vi "Get RLC Circuit Frequency Responce.vi"(0 "Vin amplitude":dbl=240.0 format="%0.2f", 1 "Circuit Type Enum":T2, 5 "Resistence (R)":dbl=10.0, 7 "Impedence (H)":dbl=0.01, 9 "Capacitave (F)":dbl=7.5e-06, 11 "error in (no error)":errorcluster) -> (3 "Frequency Response Picture":picture, 4 "Frequency Response Image Data":T1, 14 "Frequency Response":cluster{"X":dbl[], "Y":dbl[]}[](graph)=[{"X"=[0.0, 1.0, 2.0, 3.0, 4.0, 5.0, 6.0, 7.0, 8.0, 9.0, 10.0, 11.0, 12.0, 13.0, 14.0, 15.0, 16.0, 17.0, 18.0, 19.0, 20.0, 21.0, 22.0, 23.0, 24.0, 25.0, 26.0, 27.0, 28.0, 29.0, 30.0, 31.0, 32.0, 33.0, 34.0, 35.0, 36.0, 37.0, 38.0, 39.0, 40.0, 41.0, 42.0, 43.0, 44.0, 45.0, 46.0, 47.0, 48.0, 49.0, 50.0, 51.0, 52.0, 53.0, 54.0, 55.0, 56.0, 57.0, 58.0, 59.0, 60.0, 61.0, 62.0, 63.0, 64.0, 65.0, 66.0, 67.0, 68.0, 69.0, 70.0, 71.0, 72.0, 73.0, 74.0, 75.0, 76.0, 77.0], "Y"=[0.0, 0.0001279093439907941, 0.0005116286274565821, 0.0011511316053372826, 0.002046374537398417, 0.003197296190529561, 0.004603817841962096, 0.006265843283406199, 0.008183258826106956, 0.010355933306819496, 0.012783718094703, 0.01546644709913344, 0.018403936778434823, 0.0215959861495288, 0.025042376798502308, 0.028742872892093246, 0.0326972211900935, 0.036905151058669455, 0.04136637448459942, 0.04608058609042774, 0.05104746315053532, 0.05626666560812573, 0.061737836093127274, 0.06746059994101006, 0.07343456521251747, 0.07965932271431238, 0.08613444602053646, 0.09285949149528333, 0.09983399831598429, 0.10705748849770579, 0.11452946691835893, 0.12224942134482022, 0.13021682245996197, 0.13843112389059317, 0.14689176223630918, 0.1555981570992499, 0.164549711114766, 0.17374580998299163, 0.18318582250132406, 0.19286910059780862, 0.2027949793654282, 0.21296277709729705, 0.22337179532275803, 0.2340213188443811, 0.24491061577586495, 0.2560389375808376, 0.2674055191125576, 0.279009578654514, 0.2908503179619234, 0.3029269223041252, 0.3152385605078709, 0.3277843850015102, 0.3405635318600694, 0.35357512085122345, 0.36681825548215957, 0.38029202304733173, 0.39399549467710293, 0.40792772538727934, 0.4220877541295284, 0.43647460384268355, 0.4510872815049364, 0.46592477818690975, 0.48098606910561315, 0.49627011367928237, 0.5117758555830951, 0.5275022228057681, 0.5434481277070307, 0.5596124670759731, 0.5759941221902721, 0.5925919588762874, 0.6094048275700303, 0.6264315633790047, 0.6436709861449139, 0.6611219005072388, 0.6787830959676776, 0.6966533469554558, 0.7147314128934922, 0.7330160382654349]}, {"X"=[581.1516831325472, 581.1516831325472, 581.1516831325472, 581.1516831325472, 581.1516831325472, 581.1516831325472, 581.1516831325472, 581.1516831325472, 581.1516831325472, 581.1516831325472, 581.1516831325472, 581.1516831325472, 581.1516831325472, 581.1516831325472, 581.1516831325472, 581.1516831325472, 581.1516831325472, 581.1516831325472, 581.1516831325472, 581.1516831325472, 581.1516831325472, 581.1516831325472, 581.1516831325472, 581.1516831325472, 581.1516831325472, 581.1516831325472, 581.1516831325472, 581.1516831325472, 581.1516831325472, 581.1516831325472, 581.1516831325472, 581.1516831325472, 581.1516831325472, 581.1516831325472, 581.1516831325472, 581.1516831325472, 581.1516831325472, 581.1516831325472, 581.1516831325472, 581.1516831325472, 581.1516831325472, 581.1516831325472, 581.1516831325472, 581.1516831325472, 581.1516831325472, 581.1516831325472, 581.1516831325472, 581.1516831325472, 581.1516831325472, 581.1516831325472, 581.1516831325472, 581.1516831325472, 581.1516831325472, 581.1516831325472, 581.1516831325472, 581.1516831325472, 581.1516831325472, 581.1516831325472, 581.1516831325472, 581.1516831325472, 581.1516831325472, 581.1516831325472, 581.1516831325472, 581.1516831325472, 581.1516831325472, 581.1516831325472, 581.1516831325472, 581.1516831325472, 581.1516831325472, 581.1516831325472, 581.1516831325472, 581.1516831325472, 581.1516831325472, 581.1516831325472, 581.1516831325472, 581.1516831325472, 581.1516831325472, 581.1516831325472], "Y"=[0.0, 0.0, 0.0, 0.0, 0.0, 0.0, 0.0, 0.0, 0.0, 0.0, 0.0, 0.0, 0.0, 0.0, 0.0, 0.0, 0.0, 0.0, 0.0, 0.0, 0.0, 0.0, 0.0, 0.0, 0.0, 0.0, 0.0, 0.0, 0.0, 0.0, 0.0, 0.0, 0.0, 0.0, 0.0, 0.0, 0.0, 0.0, 0.0, 0.0, 0.0, 0.0, 0.0, 0.0, 0.0, 0.0, 0.0, 0.0, 0.0, 0.0, 0.0, 0.0, 0.0, 0.0, 0.0, 0.0, 0.0, 0.0, 0.0, 0.0, 0.0, 0.0, 0.0, 0.0, 0.0, 0.0, 0.0, 0.0, 0.0, 0.0, 0.0, 0.0, 0.0, 0.0, 0.0, 0.0, 0.0, 0.0]}, {"X"=[290.5758415662736, 290.5758415662736, 290.5758415662736, 290.5758415662736, 290.5758415662736, 290.5758415662736, 290.5758415662736, 290.5758415662736, 290.5758415662736, 290.5758415662736, 290.5758415662736, 290.5758415662736, 290.5758415662736, 290.5758415662736, 290.5758415662736, 290.5758415662736, 290.5758415662736, 290.5758415662736, 290.5758415662736, 290.5758415662736, 290.5758415662736, 290.5758415662736, 290.5758415662736, 290.5758415662736, 290.5758415662736, 290.5758415662736, 290.5758415662736, 290.5758415662736, 290.5758415662736, 290.5758415662736, 290.5758415662736, 290.5758415662736, 290.5758415662736, 290.5758415662736, 290.5758415662736, 290.5758415662736, 290.5758415662736, 290.5758415662736, 290.5758415662736, 290.5758415662736, 290.5758415662736, 290.5758415662736, 290.5758415662736, 290.5758415662736, 290.5758415662736, 290.5758415662736, 290.5758415662736, 290.5758415662736, 290.5758415662736, 290.5758415662736, 290.5758415662736, 290.5758415662736, 290.5758415662736, 290.5758415662736, 290.5758415662736, 290.5758415662736, 290.5758415662736, 290.5758415662736, 290.5758415662736, 290.5758415662736, 290.5758415662736, 290.5758415662736, 290.5758415662736, 290.5758415662736, 290.5758415662736, 290.5758415662736, 290.5758415662736, 290.5758415662736, 290.5758415662736, 290.5758415662736, 290.5758415662736, 290.5758415662736, 290.5758415662736, 290.5758415662736, 290.5758415662736, 290.5758415662736, 290.5758415662736, 290.5758415662736], "Y"=[0.0, 0.0, 0.0, 0.0, 0.0, 0.0, 0.0, 0.0, 0.0, 0.0, 0.0, 0.0, 0.0, 0.0, 0.0, 0.0, 0.0, 0.0, 0.0, 0.0, 0.0, 0.0, 0.0, 0.0, 0.0, 0.0, 0.0, 0.0, 0.0, 0.0, 0.0, 0.0, 0.0, 0.0, 0.0, 0.0, 0.0, 0.0, 0.0, 0.0, 0.0, 0.0, 0.0, 0.0, 0.0, 0.0, 0.0, 0.0, 0.0, 0.0, 0.0, 0.0, 0.0, 0.0, 0.0, 0.0, 0.0, 0.0, 0.0, 0.0, 0.0, 0.0, 0.0, 0.0, 0.0, 0.0, 0.0, 0.0, 0.0, 0.0, 0.0, 0.0, 0.0, 0.0, 0.0, 0.0, 0.0, 0.0]}, {"X"=[871.7275246988208, 871.7275246988208, 871.7275246988208, 871.7275246988208, 871.7275246988208, 871.7275246988208, 871.7275246988208, 871.7275246988208, 871.7275246988208, 871.7275246988208, 871.7275246988208, 871.7275246988208, 871.7275246988208, 871.7275246988208, 871.7275246988208, 871.7275246988208, 871.7275246988208, 871.7275246988208, 871.7275246988208, 871.7275246988208, 871.7275246988208, 871.7275246988208, 871.7275246988208, 871.7275246988208, 871.7275246988208, 871.7275246988208, 871.7275246988208, 871.7275246988208, 871.7275246988208, 871.7275246988208, 871.7275246988208, 871.7275246988208, 871.7275246988208, 871.7275246988208, 871.7275246988208, 871.7275246988208, 871.7275246988208, 871.7275246988208, 871.7275246988208, 871.7275246988208, 871.7275246988208, 871.7275246988208, 871.7275246988208, 871.7275246988208, 871.7275246988208, 871.7275246988208, 871.7275246988208, 871.7275246988208, 871.7275246988208, 871.7275246988208, 871.7275246988208, 871.7275246988208, 871.7275246988208, 871.7275246988208, 871.7275246988208, 871.7275246988208, 871.7275246988208, 871.7275246988208, 871.7275246988208, 871.7275246988208, 871.7275246988208, 871.7275246988208, 871.7275246988208, 871.7275246988208, 871.7275246988208, 871.7275246988208, 871.7275246988208, 871.7275246988208, 871.7275246988208, 871.7275246988208, 871.7275246988208, 871.7275246988208, 871.7275246988208, 871.7275246988208, 871.7275246988208, 871.7275246988208, 871.7275246988208, 871.7275246988208], "Y"=[0.0, 0.0, 0.0, 0.0, 0.0, 0.0, 0.0, 0.0, 0.0, 0.0, 0.0, 0.0, 0.0, 0.0, 0.0, 0.0, 0.0, 0.0, 0.0, 0.0, 0.0, 0.0, 0.0, 0.0, 0.0, 0.0, 0.0, 0.0, 0.0, 0.0, 0.0, 0.0, 0.0, 0.0, 0.0, 0.0, 0.0, 0.0, 0.0, 0.0, 0.0, 0.0, 0.0, 0.0, 0.0, 0.0, 0.0, 0.0, 0.0, 0.0, 0.0, 0.0, 0.0, 0.0, 0.0, 0.0, 0.0, 0.0, 0.0, 0.0, 0.0, 0.0, 0.0, 0.0, 0.0, 0.0, 0.0, 0.0, 0.0, 0.0, 0.0, 0.0, 0.0, 0.0, 0.0, 0.0, 0.0, 0.0]}] caption="XY Graph", 15 "error out":errorcluster)   [LabVIEW 2017]
uses:
  Types/Circuit Type Enum.ctl
  <vilib>/picture/picture.llb/imagedata.ctl
panel:
  out "Frequency (H)":dbl(slide)=77.0 scale=0.0..3000.0
  out "XL":dbl=4.838052686528282
  out "Xc":dbl=275.59297505090103
  out "Supply Current (A)":dbl(slide)=0.7330160382654349 scale=0.0..100.0
  out "Fo":dbl=581.1516831325472
  out "Fl":dbl=290.5758415662736
  out "Fh":dbl=871.7275246988208
  out "Half Band":dbl=290.5758415662736
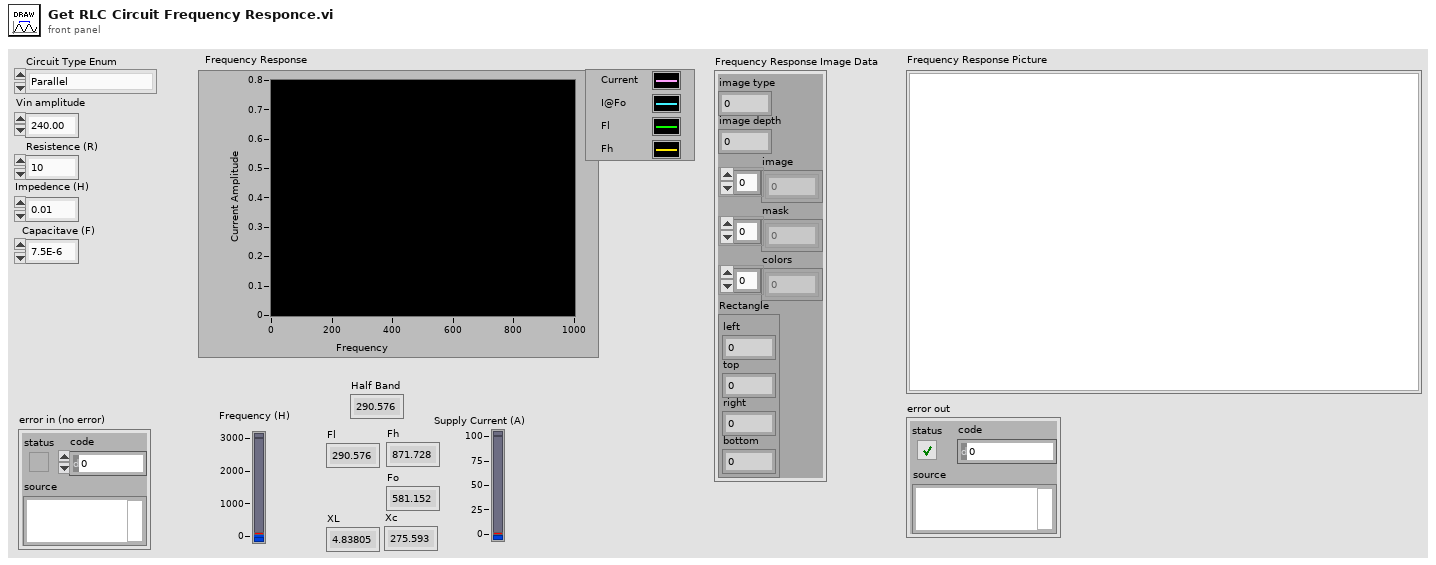
[diagram p1: front panel]
types:
  T1 = typedef "imagedata.ctl" = cluster{"image type":i32, "image depth":i32, "image":u8[], "mask":u8[], "colors":u32[], "Rectangle":cluster{"left":i16, "top":i16, "right":i16, "bottom":i16}}
  T2 = typedef "Circuit Type Enum.ctl" = enum16{"Parallel", "Serial"}
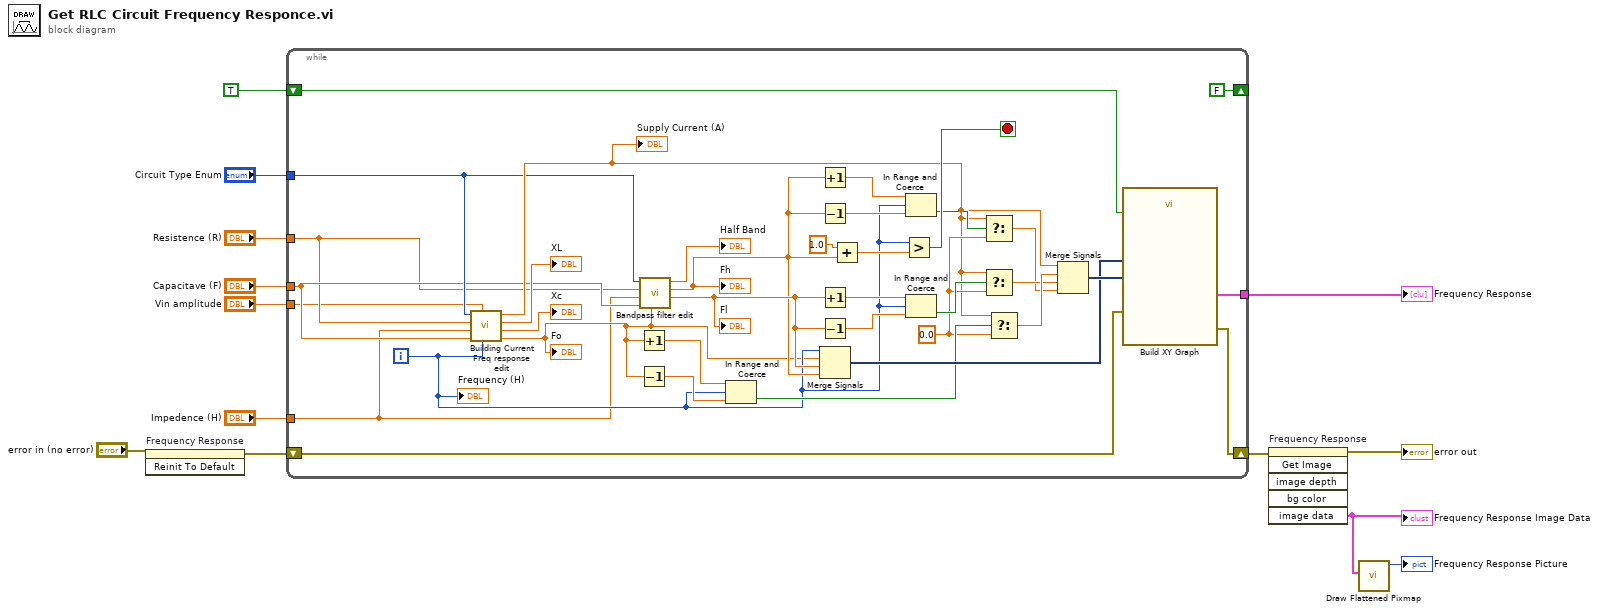
[diagram p0: block diagram]
diagram:
  n1 = invoke on="Frequency Response" class="XYGraph (strict)" method="Reinit To Default"(error in="error in (no error)") -> (error out=w3:errorcluster)  [unwired: 2 in, 2 out]
  n2 = while {
    tunnel: "Circuit Type Enum" -> [w23]
    tunnel: "Capacitave (F)" -> [w22]
    tunnel: "Resistence (R)" -> [w21]
    tunnel: "Vin amplitude" -> [w20]
    tunnel: "Impedence (H)" -> [w19]
    tunnel: [w18] -> w8
    shift-right: [w16] -> w7
    shift-left: w3 -> [w17]
    shift-right: [FALSE] -> _
    shift-left: TRUE -> [w15]
    i -> [w25]
    stop <- w47 stop-if-true
    w33 = 0.0 ("f")
    n3 = call "Building Current Freq response edit.vi"("F variable"=w25, "Vin"=w20, "C"=w22, "L"=w19, "R"=w21, "Circuit Type Enum"=w23) -> ("Fo"=w24:dbl, "Xc"=→"Xc":dbl, "Xl"=→"XL":dbl, "Supply Current"=w31:dbl)  [unwired: 2 in]
    "Supply Current (A)" <- w31
    "Fo" <- w24
    n4 = Increment(x=w24) -> (x+1=w41:dbl)
    n5 = Decrement(x=w24) -> (x-1=w46:dbl)
    n6 = call "Bandpass filter edit.vi"("Fr"=w24, "C"=w22, "L"=w19, "R"=w21, "Circuit Type"=w23) -> ("Fl"=w28:dbl, "Fh"=w27:dbl, "half"=→"Half Band":dbl)  [unwired: 4 in]
    "Fl" <- w28
    "Fh" <- w27
    n7 = In Range and Coerce(upper limit=w41, x=w25, lower limit=w46) -> (In Range?=w45:bool)  [unwired: 1 out]
    n8 = Increment(x=w27) -> (x+1=w36:dbl)
    n9 = Decrement(x=w27) -> (x-1=w35:dbl)
    n10 = Increment(x=w28) -> (x+1=w40:dbl)
    n11 = Decrement(x=w28) -> (x-1=w39:dbl)
    n12 = Merge Signals(w25, w24, w28, w27) -> (w48:dynamicdata)
    n13 = Add(x=1.0, y=w27) -> (x+y=w43:dbl)
    n14 = Greater?(x=w25, y=w43) -> (0:w47:bool)
    n15 = In Range and Coerce(upper limit=w36, x=w25, lower limit=w35) -> (In Range?=w34:bool)  [unwired: 1 out]
    n16 = In Range and Coerce(upper limit=w40, x=w25, lower limit=w39) -> (In Range?=w38:bool)  [unwired: 1 out]
    n17 = Select(t=w31, s=w34, f=w33) -> (s? t:f=w32:dbl)
    n18 = Select(t=w31, s=w38, f=w33) -> (s? t:f=w37:dbl)
    n19 = Select(t=w31, s=w45, f=w33) -> (s? t:f=w44:dbl)
    n20 = Merge Signals(w31, w44, w37, w32) -> (w49:dynamicdata)
    n21 = call "Build XY Graph"("error in (no error)"=w17, "Reset"=w15, "Y Input"=w49, "X Input"=w48) -> ("error out"=w16:errorcluster, "XY Graph"=w18:cluster{"X":dbl[], "Y":dbl[]}[])  [unwired: 6 in]
    "Frequency (H)" <- w25
  }
  "Frequency Response" <- w8
  n22 = invoke on="Frequency Response" class="XYGraph (strict)" method="Get Image"(error in=w7) -> (error out=→"error out":errorcluster, "image data"=w5:T1)  [unwired: 5 in, 4 out]
  "Frequency Response Image Data" <- w5
  n23 = call <vilib>:"Draw Flattened Pixmap.vi"("image data"=w5) -> ("new picture"=→"Frequency Response Picture":picture)  [unwired: 8 in]
